vi "Example - Monitoring_receiver_v0.1.vi"() -> ()   [LabVIEW 2015, in "Monitoring_receiver.lvlib"]
uses:
  Monitoring_receiver.lvlib
  <vilib>/userdefined/High Color/nirio_resource_hc.ctl
  Proto/Host_Simple/Typedef/ChannelSelector_cluster.ctl
  <vilib>/FPGAPlugInAG/PXIe-7965R/niLvFpga_Open_PXIe-7965R.vi
  <vilib>/rvi/interface/common/dynamic/niFpgaDynamicAddResources.vi
  <vilib>/Utility/error.llb/Error Cluster From Error Code.vi
  <vilib>/rvi/errors/niLvFpgaAdjustHostInterfaceError.vi
  <vilib>/FPGAPlugInAG/Dynamic/niLvFpga_Close_Dynamic.vi
  <vilib>/rvi/interface/nirviOpenFPGA/nirviOpenFPGA.xnode
  FPGA Bitfiles/DDC_FPGATarget_DDCmain0v9_166F806D.lvbitx
  <vilib>/rvi/interface/nirviReadWriteControl/nirviReadWriteControl.xnode
  <vilib>/rvi/interface/nirviCloseFPGA/nirviCloseFPGA.xnode
  <vilib>/rvi/interface/Simulation/niFpgaSimulationCallBeginRW.vi
  NiFpgaLv.dll
panel:
  out "max value":i16
  in  "Enable Sw DDC":bool=TRUE
  in  "length":i32(slide) scale=0.0..65535.0
  in  "index":i32(slide) scale=0.0..100000.0
  in  "passband bandwidth (Hz)":dbl format="%.2p"
  in  "carrier frequency (Hz)":dbl min=-0.5 max=0.5 format="%.2p"
  out "cmd.received":string
  in  "Client Closed 2":string="The client VI closed the connection."
  out "cmd.server.ready":bool caption="TCP Cmd Srv Rdy"
  out "data.server.ready":bool caption="TCP Data Srv Rdy"
  in  "Client Closed":string="The client VI closed the connection."
  in  "Channels":T1={"RIO0"=[[TRUE, TRUE]], "RIO1"=[]} caption="Channel selector"
  out "Power Spectrum":cluster{"f0":dbl, "df":dbl, "magnitude":dbl[]}[](graph)
  out "DDCRunnig":bool=TRUE
  in  "Debug info":bool
  out "Tab Control":enum32{"Debug On", "Debug Off"}(tab)
  out "Data in size":i32[](array[numeric])
  in  "Phase offset":dbl
  out "Trigger Pressed?":bool
  out "DMA Remaining":u32[](array[numeric])
  out "error out":errorcluster
  out "CountFIFOout":u32
  out "CountCIC2out":u32
  out "CountFIR2out":u32
  out "Remaining1":u32[](array[numeric])
  out "Remaining2":u32[](array[numeric])
  out "DMA \nTimed out":bool[](array[boolean])
  out "Device\nConfigured":bool[](array[boolean])
  in  "Resources":T2[](array[typedef])=["PXI1Slot12"]
  in  "Poff_Simulated":fxp<+,32,32> caption="Phase Offset"
  in  "Acq Time (ms)":u64=10
  in  "Continuous Acquisition":bool=TRUE
  in  "Software Trigger":bool
  in  "fLO (MHz)":dbl=36.0 caption="DDS Frequency (MHz)" format="%.6f"
  in  "Amplitude scale":fxp<+,20,16>=4000.0
  in  "f_Synth (MHz)":dbl=10.0 caption="Frequency (MHz) (MHz)" format="%#.7f"
  in  "Mode":enum16{"Real IO", "Constant", "Simulated"}(ring)
  out "Analog Input":waveform(dbl)[](graph) caption="Waveform"
  in  "stop":bool
  # "Digital Receiver Demo - NI 5772"
  # "Ver 2.27.0 , © Peter Vago, NI SE , 2017"
  # "Resources"
  # "Direct Digital Receiver"
  # "Simulation Signal Generator"
  # "RIO0"
  # "Ch2\n Ch3"
  # "RIO1"
  # "Debug Info"
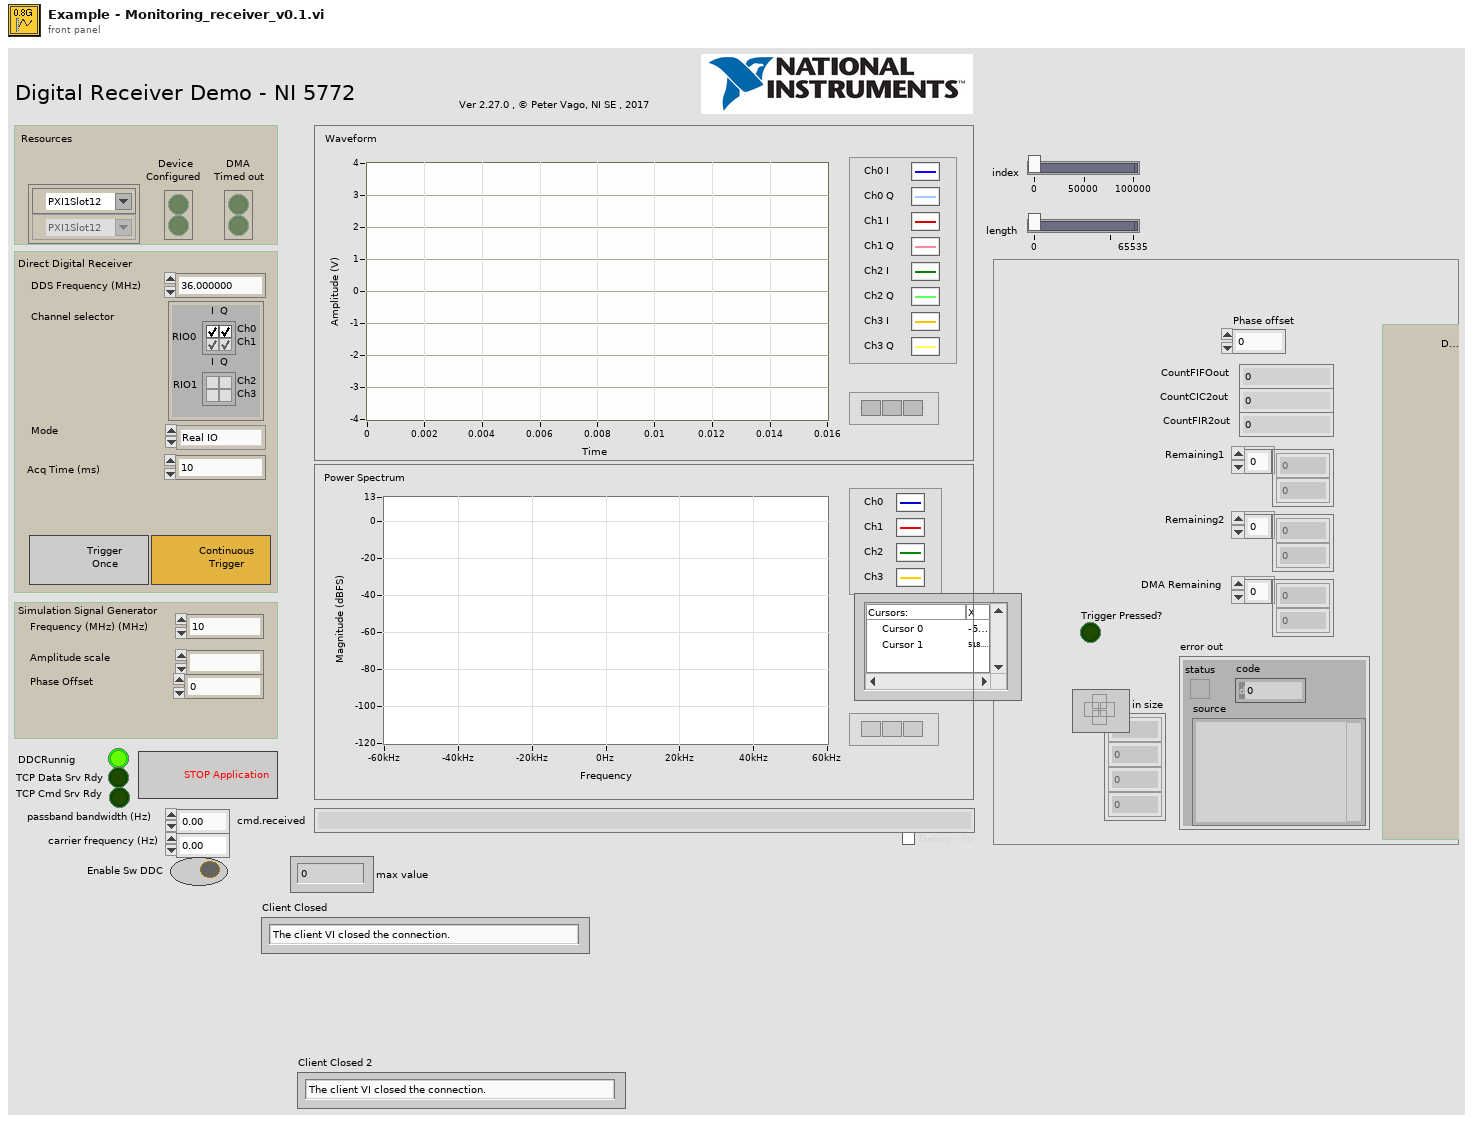
[diagram p1: front panel]
types:
  T1 = typedef "ChannelSelector_cluster.ctl" = cluster{"RIO0":bool[][], "RIO1":bool[][]}
  T2 = typedef "nirio_resource_hc.ctl" = tag
  T3 = enum8{"Internal Clock PLL Off", "Internal Clock PLL On (REF IN)", "External Clock (CLK_IN)", "Internal Clock PLL On (IoModSyncClk)"}
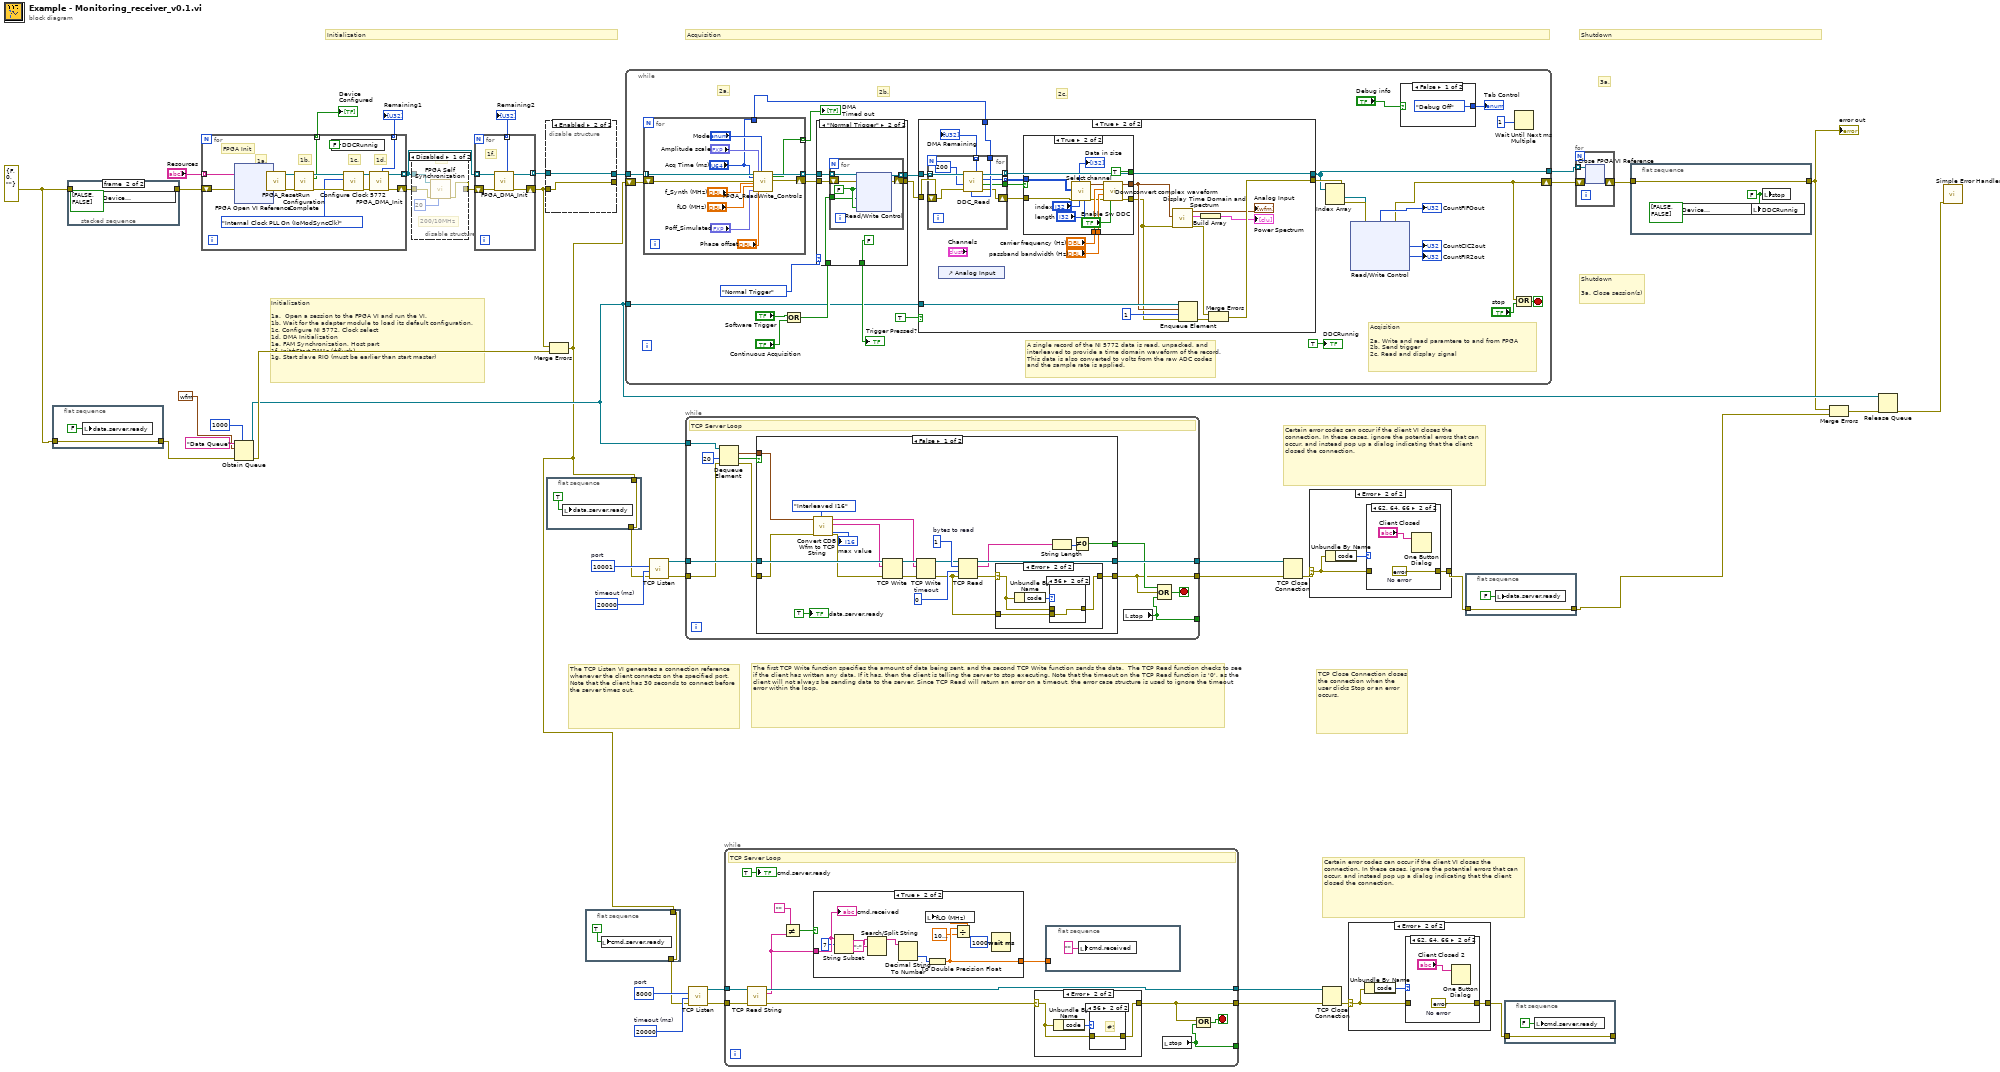
[diagram p0: block diagram]
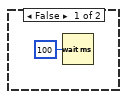
[diagram p4: hidden frame]
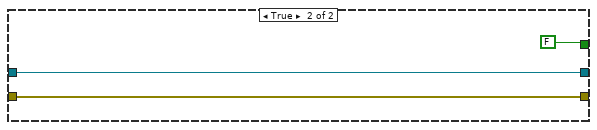
[diagram p11: hidden frame]
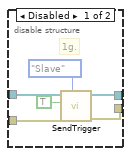
[diagram p13: hidden frame]
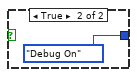
[diagram p15: hidden frame]
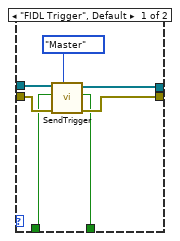
[diagram p16: hidden frame]
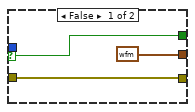
[diagram p18: hidden frame]
diagram:
  w5 = u16 8000  # port
  w6 = 20000  # timeout (ms)
  w14 = u16 10001  # port
  w15 = 20000  # timeout (ms)
  w23 = errorcluster {"status"=FALSE, "code"=0, "source"=""} ("error out")
  # "Certain error codes can occur if the client VI closes the connection. In these cases, ignore the potential errors that can occur, and instead pop up a dialog indicating that the client closed the connection."
  # "Certain error codes can occur if the client VI closes the connection. In these cases, ignore the potential errors that can occur, and instead pop up a dialog indicating that the client closed the connection."
  # "TCP Close Connection closes the connection when the user clicks Stop or an error occurs."
  # "The TCP Listen VI generates a connection reference whenever the client connects on the specified port. Note that the client has 30 seconds to connect before the server times out."
  # "The first TCP Write function specifies the amount of data being sent, and the second TCP Write function sends the data.  The TCP Read function checks to see if the client has written any data. If it has, then the client is telling the server to stop executing. Note that the timeout on the TCP Read function is '0', as the client will not always be sending data to the server. Since TCP Read will return an error on a timeout, the error case structure is used to ignore the timeout error within the loop."
  # "Shutdown\n\n3a. Close session(s)"
  # "3a."
  # "Acquisition"
  # "Shutdown"
  # "Initialization\n\n1a.  Open a session to the FPGA VI and run the VI.\n1b. Wait for the adapter module to load its default configuration.\n1c. Configure NI 5772, Clock select\n1d. DMA Initialization\n1e. FAM Synchronization, Host part\n1f. Init+Start DMAs (+flush)\n1g. Start slave RIO (must be earlier than start master)"
  # "Initialization"
  n1 = flat-sequence {
    tunnel: w23 -> [w45]
    tunnel: [w45] -> w22
    frame #0 {
      n2 = local write "data.server.ready"(FALSE ("data.server.ready")) -> ()
    }
  }
  n3 = stacked-sequence {
    tunnel: [w47 _] -> w34
    tunnel: w23 -> [w47 _]
    frame #0 {
    }
    frame #1 {
      n4 = local write "Device\nConfigured"(bool[] [FALSE, FALSE] ("Configured?")) -> ()
    }
  }
  n5 = for {
    tunnel: [w64] -> w37 mode=indexing
    tunnel: "Resources" -> [w53] mode=indexing
    shift-right: [w63] -> w40
    shift-left: w34 -> [w52]
    tunnel: [w51] -> w41 mode=indexing
    tunnel: [w49] -> w38 mode=indexing
    # "1d."
    # "1c."
    # "FPGA Init"
    # "1b."
    # "1a."
    n6 = xnode "FPGA Open VI Reference"("error in"=w52, "resource name"=w53) -> ("FPGA VI Reference Out"=w62:refnum<k20>, "error out"=w55:errorcluster)
    n7 = call "FPGA_ResetRun.vi"("error in (no error)"=w55, "Refnum in"=w62) -> ("error out"=w54:errorcluster, "Refnum out"=w61:refnum<k20>)  [unwired: 8 in]
    n8 = call "Configuration Complete.vi"("error in"=w54, "FPGA VI Reference In"=w61) -> ("error out"=w58:errorcluster, "Configured?"=w51:bool, "FPGA VI Reference Out"=w60:refnum<k20>)  [unwired: 7 out]
    n9 = local write "DDCRunnig"(FALSE ("Run")) -> ()
    n10 = call "Configure Clock 5772.vi"("error in"=w58, "Clock Source"=T3."Internal Clock PLL On (IoModSyncClk)", "FPGA VI Reference In"=w60) -> ("error out"=w57:errorcluster, "FPGA VI Reference Out"=w59:refnum<k20>)  [unwired: 6 in, 1 out]
    n11 = call "FPGA_DMA_Init.vi"("error in (no error)"=w57, "Refnum in"=w59) -> ("error out"=w63:errorcluster, "Refnum out"=w64:refnum<k20>, "Remaining"=w49:u32)  [unwired: 7 in]
  }
  "Device\nConfigured" <- w41
  "Remaining1" <- w38
  n12 = Obtain Queue(max queue size (-1, unlimited)=1000, name (unnamed)="Data Queue", element data type=waveform(cdb) {"t0"=timestamp(0 s since 1904-01-01), "dt"=1.0, "Y"=[]} ("output waveform"), error in (no error)=w22) -> (queue out=w27:refnum<queue>, error out=w29:errorcluster)  [unwired: 1 in, 1 out]
  n13 = disable-structure shown="Disabled" {
    disable-tunnel: w40 -> [w68 w69]
    disable-tunnel: w37 -> [w66 _]
    disable-tunnel: [w65 w69] -> w36
    frame Disabled {
      # "1e."
      # "200/10MHz"
      n14 = call <instrlib>:"FPGA Self Synchronization.vi"("sync.cptr.Period"=u16 20, "error in"=w68, "FPGA VI References In"=w66) -> ("error out"=w65:errorcluster)  [unwired: 7 in, 1 out]
    }
    frame Enabled {
    }
  }
  n15 = for {
    tunnel: w37 -> [w72] mode=indexing
    tunnel: [w71] -> w33 mode=indexing
    shift-right: [w73] -> w28
    shift-left: w36 -> [w74]
    tunnel: [w70] -> w35 mode=indexing
    # "1f."
    n16 = call "FPGA_DMA_Init.vi"("error in (no error)"=w74, "Refnum in"=w72) -> ("error out"=w73:errorcluster, "Refnum out"=w71:refnum<k20>, "Remaining"=w70:u32)  [unwired: 7 in]
  }
  "Remaining2" <- w35
  n17 = disable-structure shown="Enabled" {
    disable-tunnel: w33 -> [w80 w82]
    disable-tunnel: [w79 w82] -> w32
    disable-tunnel: w28 -> [w77 w81]
    disable-tunnel: [w76 w81] -> _
    frame Disabled {
      # "1g."
      n18 = call "SendTrigger.vi"("Master/Slave"=enum16{"Master", "Slave"}."Slave", "error in (no error)"=w77, "Trigger in"=TRUE, "Resources in"=w80) -> ("error out"=w76:errorcluster, "Resources out"=w79:refnum<k20>[])  [unwired: 5 in, 1 out]
    }
    frame Enabled {
    }
  }
  n19 = flat-sequence {
    tunnel: w2 -> [w83]
    tunnel: [w83] -> w12
    frame #0 {
      n20 = local write "data.server.ready"(TRUE ("data.server.ready")) -> ()
    }
  }
  n21 = Merge Errors(w28, w29) -> (w2:errorcluster)
  n22 = flat-sequence {
    tunnel: w2 -> [w85]
    tunnel: [w85] -> w3
    frame #0 {
      n23 = local write "cmd.server.ready"(TRUE ("data.server.ready")) -> ()
    }
  }
  n24 = while {
    shift-right: [w87] -> w44
    shift-left: w2 -> [w112]
    tunnel: w32 -> [w107]
    tunnel: [w96] -> w39
    tunnel: w27 -> [w90]
    stop <- w113 stop-if-true
    # "Acqisition\n\n2a. Write and read paramtere to and from FPGA\n2b. Send trigger\n2c. Read and display signal"
    # "2c."
    # "2b."
    # "2a."
    # "A single record of the NI 5772 data is read, unpacked, and interleaved to provide a time domain waveform of the record. This data is also converted to volts from the raw ADC codes and the sample rate is applied."
    n25 = for {
      tunnel: w107 -> [w147] mode=indexing
      shift-right: [w144] -> w105
      shift-left: w112 -> [w145]
      tunnel: [w146] -> w102 mode=indexing
      tunnel: [w138] -> w106 mode=indexing
      tunnel: ["Acq Time (ms)"] -> w89
      n26 = call "FPGA_ReadWrite_Controls.vi"("Refnum in"=w147, "Acq Time (ms)"="Acq Time (ms)", "error in (no error)"=w145, "f_Synth (MHz)"="f_Synth (MHz)", "fLO (MHz)"="fLO (MHz)", "Poff_Simulated"="Poff_Simulated", "Scale Synth"="Amplitude scale", "Phase offset"="Phase offset", "Mode"="Mode") -> ("Refnum out"=w146:refnum<k20>, "DMA Timed Out?"=w138:bool, "error out"=w144:errorcluster)  [unwired: 4 in, 4 out]
    }
    "DMA \nTimed out" <- w106
    n27 = Or(x="Software Trigger", y="Continuous Acquisition") -> (x .or. y?=w101:bool)
    n28 = case shown="\"Normal Trigger\"" enum16{"FIDL Trigger", "Normal Trigger"}."Normal Trigger" {
      tunnel: w105 -> [w123 w128]
      tunnel: [w122 w129] -> w103
      tunnel: w102 -> [w120 w127]
      tunnel: [w117 w126] -> w100
      tunnel: w101 -> [w121 w125]
      tunnel: [w118 FALSE ("Trigger Pressed?")] -> w91
      frame "FIDL Trigger", Default {
        n29 = call "SendTrigger.vi"("Master/Slave"=enum16{"Master", "Slave"}."Master", "error in (no error)"=w123, "Trigger in"=w121, "Resources in"=w120) -> ("error out"=w122:errorcluster, "Trigger Pressed?"=w118:bool, "Resources out"=w117:refnum<k20>[])  [unwired: 5 in]
      }
      frame "Normal Trigger" {
        n30 = for {
          shift-right: [w134] -> w129
          shift-left: w128 -> [w133]
          tunnel: w127 -> [w132] mode=indexing
          tunnel: [w131] -> w126 mode=indexing
          tunnel: w125 -> [w130]
          w135 = FALSE
          n31 = xnode "Read/Write Control"("FPGA VI Reference In"=w132, "error in"=w133, "Trigger"=w135, "Trigger"=w130, "Trigger"=w135) -> ("FPGA VI Reference Out"=w131:refnum<k20>, "error out"=w134:errorcluster)
        }
      }
    }
    "Trigger Pressed?" <- w91
    n32 = case shown="True" TRUE {
      tunnel: [w148 w158] -> w108
      tunnel: [w149 w169] -> w96
      tunnel: w100 -> [w149 w168]
      tunnel: w103 -> [w148 w167]
      tunnel: w90 -> [_ w164]
      tunnel: w89 -> [_ w157]
      frame False {
      }
      frame True {
        n33 = for {
          tunnel: [w193] -> w169 mode=indexing
          tunnel: w168 -> [w192] mode=indexing
          shift-right: [w186] -> w162
          shift-left: w167 -> [w188]
          tunnel: [w191] -> w166 mode=indexing
          tunnel: [w187] -> w165 mode=indexing
          tunnel: w157 -> [w190]
          tunnel: [w185] -> w156
          n34 = call "DDC_Read.vi"("milliseconds to wait"=w190, "error in (no error)"=w188, "ms to read"=200, "Refnum in"=w192) -> ("error out"=w186:errorcluster, "Output valid"=w185:bool, "Data"=w187:u64[], "Refnum out"=w193:refnum<k20>, "Elements Remaining"=w191:u32)  [unwired: 3 in]
        }
        "DMA Remaining" <- w166
        n35 = control-ref of="Analog Input"() -> ()  [unwired: 1 out]
        n36 = case shown="True" w156 {
          selector: w156 -> [w170 _]
          tunnel: w165 -> [_ w181]
          tunnel: w162 -> [w172 w179]
          tunnel: "carrier frequency (Hz)" -> [_ w184]
          tunnel: "passband bandwidth (Hz)" -> [_ w183]
          tunnel: [w172 w182] -> w151
          tunnel: [waveform(cdb) {"t0"=timestamp(0 s since 1904-01-01), "dt"=1.0, "Y"=[]} ("output waveform out") w177] -> w152
          tunnel: [w170 TRUE] -> _
          frame False {
          }
          frame True {
            n37 = call "Select channel.vi"("length"="length", "index"="index", "err in"=w179, "Data in"=w181) -> ("output waveform"=w178:waveform(cdb), "Data in size"=→"Data in size":i32[])  [unwired: 5 in, 1 out]
            n38 = call "Downconvert complex waveform.vi"("Enable Sw DDC"="Enable Sw DDC", "error in (no error)"=w179, "passband bandwidth (Hz)"=w183, "carrier frequency (Hz)"=w184, "CDB Wfm in"=w178) -> ("error out"=w182:errorcluster, "output waveform out"=w177:waveform(cdb))  [unwired: 5 in]
          }
        }
        n39 = call "Display Time Domain and Spectrum.vi"("error in (no error)"=w151, "CDB Wfm in"=w152) -> ("error out"=w150:errorcluster, "Power Spectrum / PSD"=w154:cluster{"f0":dbl, "df":dbl, "magnitude":dbl[]}, "I and Q Waveform"=→"Analog Input":waveform(dbl)[])  [unwired: 7 in]
        n40 = Enqueue Element(queue=w164, element=w152, timeout in ms (-1)=1, error in (no error)=w151) -> (error out=w159:errorcluster)  [unwired: 2 out]
        n41 = Build Array(w154) -> (→"Power Spectrum":cluster{"f0":dbl, "df":dbl, "magnitude":dbl[]}[])
        n42 = Merge Errors(w150, w159) -> (w158:errorcluster)
      }
    }
    n43 = Index Array(array=w96) -> (element #1=w95:refnum<k20>)  [unwired: 2 in, 1 out]
    n44 = xnode "Read/Write Control"("FPGA VI Reference In"=w95, "error in"=w108) -> ("error out"=w87:errorcluster, "CountFIFO"=→"CountFIFOout":u32, "CountCIC2out"=→"CountCIC2out":u32, "CountFIR2out"=→"CountFIR2out":u32)  [unwired: 1 in, 1 out]
    n45 = case shown="False" "Debug info" {
      tunnel: [enum32{"Debug On", "Debug Off"}."Debug Off" ("Tab Control") enum32{"Debug On", "Debug Off"}."Debug On" ("Tab Control")] -> w93
      frame False {
      }
      frame True {
      }
    }
    "Tab Control" <- w93
    n46 = Wait Until Next ms Multiple(millisecond multiple=u32 1 ("milliseconds to wait")) -> ()  [unwired: 1 out]
    n47 = Compound Arithmetic op=OR(w87, "stop") -> (w113:bool)
    "DDCRunnig" <- TRUE ("Run")
  }
  n48 = call <vilib>:"TCP Listen.vi"("error in (no error)"=w12, "timeout ms (wait forever: -1)"=w15, "port"=w14) -> ("error out"=w16:errorcluster, "connection ID"=w17:refnum<k5>)  [unwired: 4 in, 3 out]
  n49 = while {
    tunnel: [w201] -> w19
    tunnel: [w203] -> w20
    tunnel: w17 -> [w205]
    tunnel: w16 -> [w199]
    tunnel: w27 -> [w200]
    tunnel: [w194] -> _
    stop <- w204 stop-if-true
    # "TCP Server Loop"
    n50 = Dequeue Element(queue=w200, timeout in ms (-1)=20, error in (no error)=w199) -> (element=w195:waveform(cdb), timed out?=w197:bool, error out=w196:errorcluster)  [unwired: 1 out]
    n51 = case shown="False" w197 {
      tunnel: w205 -> [w226 w236]
      tunnel: [w219 w236] -> w203
      tunnel: [w215 FALSE] -> w202
      tunnel: [w213 w235] -> w201
      tunnel: w196 -> [w209 w235]
      tunnel: w195 -> [w210 _]
      frame False {
        w218 = 0  # timeout
        w221 = 1  # bytes to read
        n52 = call "Convert CDB Wfm to TCP String.vi"("Format (Intlvd I16)"=enum16{"Interleaved I16", "Interleaved DBL"}."Interleaved I16", "error in (no error)"=w209, "CDB Wfm in"=w210) -> ("error out"=w208:errorcluster, "Message size"=w223:string, "TCP message"=w222:string, "max value"=→"max value":i16)  [unwired: 5 in]
        n53 = TCP Write(connection ID=w226, data in=w223, error in (no error)=w208) -> (connection ID out=w225:refnum<k5>, error out=w224:errorcluster)  [unwired: 2 out]
        n54 = TCP Write(connection ID=w225, data in=w222, error in (no error)=w224) -> (connection ID out=w220:refnum<k5>, error out=w212:errorcluster)  [unwired: 2 out]
        n55 = TCP Read(connection ID=w220, bytes to read=w221, error in (no error)=w212, 9:w218) -> (connection ID out=w219:refnum<k5>, data out=w216:string, error out=w214:errorcluster)  [unwired: 1 out]
        n56 = case shown="Error" w214 {
          selector: w214 -> [w227 w230]
          tunnel: [w227 w228] -> w213
          tunnel: w212 -> [_ w229]
          frame No Error {
          }
          frame Error {
            n57 = Unbundle By Name(w230) -> ("code"=w231:i32)
            n58 = case shown="56" w231 {
              tunnel: w230 -> [w232 _]
              tunnel: w229 -> [_ w233]
              tunnel: [w232 w233] -> w228
              frame Default {
              }
              frame 56 {
              }
            }
          }
        }
        n59 = String Length(string=w216) -> (length=w217:i32)
        n60 = Not Equal To 0?(x=w217) -> (x != 0?=w215:bool)
        "data.server.ready" <- TRUE ("data.server.ready")
      }
      frame True {
      }
    }
    n61 = local read "stop"() -> (w194:bool)
    n62 = Compound Arithmetic op=OR(w202, w201, w194) -> (w204:bool)
  }
  n63 = call <vilib>:"TCP Listen.vi"("error in (no error)"=w3, "timeout ms (wait forever: -1)"=w6, "port"=w5) -> ("error out"=w7:errorcluster, "connection ID"=w8:refnum<k5>)  [unwired: 4 in, 3 out]
  n64 = while {
    tunnel: [w247] -> w10
    tunnel: [w241] -> w11
    tunnel: w8 -> [w244]
    tunnel: w7 -> [w245]
    tunnel: [w246] -> _
    stop <- w248 stop-if-true
    # "TCP Server Loop"
    n65 = call <vilib>:"TCP Read String.vi"("error in (no error)"=w245, "connection ID"=w244) -> ("error out"=w240:errorcluster, "data out"=w238:string, "connection ID out"=w241:refnum<k5>)  [unwired: 7 in]
    n66 = Not Equal?(x="", y=w238) -> (x != y?=w239:bool)
    n67 = case shown="True" w239 {
      tunnel: w238 -> [_ w260]
      tunnel: [_ w253] -> w237
      frame False {
        n68 = Wait (ms)(milliseconds to wait=u32 100) -> ()  [unwired: 1 out]
      }
      frame True {
        n69 = String Subset(string=w260, offset (0)=7) -> (substring=w258:string)  [unwired: 1 in]
        n70 = Search/Split String(string=w258, search string/char (-)=";") -> (substring before match=w256:string)  [unwired: 1 in, 2 out]
        n71 = Decimal String To Number(string=w256) -> (number=w255:i32)  [unwired: 2 in, 1 out]
        n72 = To Double Precision Float(number=w255) -> (double precision float=w253:dbl)
        n73 = Divide(x=w253, y=1000000.0) -> (x/y=w251:dbl)
        n74 = local write "fLO (MHz)"(w251) -> ()
        n75 = Wait (ms)(milliseconds to wait=u32 1000) -> ()  [unwired: 1 out]
        "cmd.received" <- w260
      }
    }
    n76 = case shown="Error" w240 {
      selector: w240 -> [w261 w263]
      tunnel: [w261 w262] -> w247
      frame No Error {
      }
      frame Error {
        n77 = Unbundle By Name(w263) -> ("code"=w264:i32)
        n78 = case shown="56" w264 {
          tunnel: w263 -> [w265 w266]
          tunnel: [w265 w266] -> w262
          frame Default {
          }
          frame 56 {
            # "#!"
          }
        }
      }
    }
    n79 = flat-sequence {
      tunnel: w237 -> [_]
      frame #0 {
        n80 = local write "cmd.received"("" ("cmd.received")) -> ()
      }
    }
    n81 = local read "stop"() -> (w246:bool)
    n82 = Compound Arithmetic op=OR(w247, w246) -> (w248:bool)
    "cmd.server.ready" <- TRUE ("data.server.ready")
  }
  n83 = TCP Close Connection(connection ID=w20, error in (no error)=w19) -> (error out=w18:errorcluster)  [unwired: 2 out]
  n84 = case shown="Error" w18 {
    selector: w18 -> [w267 w269]
    tunnel: [w267 w268] -> w13
    frame No Error {
    }
    frame Error {
      n85 = Unbundle By Name(w269) -> ("code"=w270:i32)
      n86 = case shown="62, 64, 66" w270 {
        tunnel: w269 -> [w271 _]
        tunnel: [w271 w273] -> w268
        frame Default {
        }
        frame 62, 64, 66 {
          w273 = errorcluster {"status"=FALSE, "code"=0, "source"=""}  # No error
          n87 = One Button Dialog(message="Client Closed") -> ()  [unwired: 1 in, 1 out]
        }
      }
    }
  }
  n88 = TCP Close Connection(connection ID=w11, error in (no error)=w10) -> (error out=w9:errorcluster)  [unwired: 2 out]
  n89 = case shown="Error" w9 {
    selector: w9 -> [w274 w276]
    tunnel: [w274 w275] -> w4
    frame No Error {
    }
    frame Error {
      n90 = Unbundle By Name(w276) -> ("code"=w277:i32)
      n91 = case shown="62, 64, 66" w277 {
        tunnel: w276 -> [w278 _]
        tunnel: [w278 w280] -> w275
        frame Default {
        }
        frame 62, 64, 66 {
          w280 = errorcluster {"status"=FALSE, "code"=0, "source"=""}  # No error
          n92 = One Button Dialog(message="Client Closed 2") -> ()  [unwired: 1 in, 1 out]
        }
      }
    }
  }
  n93 = flat-sequence {
    tunnel: w13 -> [w281]
    tunnel: [w281] -> w21
    frame #0 {
      n94 = local write "data.server.ready"(FALSE ("data.server.ready")) -> ()
    }
  }
  n95 = flat-sequence {
    tunnel: w4 -> [w283]
    tunnel: [w283] -> _
    frame #0 {
      n96 = local write "cmd.server.ready"(FALSE ("data.server.ready")) -> ()
    }
  }
  n97 = for {
    tunnel: w39 -> [w285] mode=indexing
    shift-right: [w286] -> w43
    shift-left: w44 -> [w287]
    n98 = xnode "Close FPGA VI Reference"("FPGA VI Reference In"=w285, "error in"=w287) -> ("error out"=w286:errorcluster)
  }
  n99 = flat-sequence {
    tunnel: w43 -> [w288]
    tunnel: [w288] -> w26
    frame #0 {
      w290 = FALSE ("stop")
      n100 = local write "Device\nConfigured"(bool[] [FALSE, FALSE] ("Configured?")) -> ()
      n101 = local write "DDCRunnig"(w290) -> ()
      n102 = local write "stop"(w290) -> ()
    }
  }
  n103 = Merge Errors(w26, w21) -> (w25:errorcluster)
  n104 = Release Queue(queue=w27, error in (no error)=w25) -> (error out=w24:errorcluster)  [unwired: 1 in, 2 out]
  n105 = call <vilib>:"Simple Error Handler.vi"("error in (no error)"=w24) -> ()  [unwired: 4 in, 5 out]
  "error out" <- w26
